vi "xboxClose.vi"() -> (0 "error out":errorcluster)   [LabVIEW 2017]
uses:
  globalDevices.vi
  <vilib>/Utility/inputDevices.llb/closeJoystick.vi
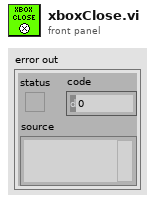
[diagram p1: front panel]
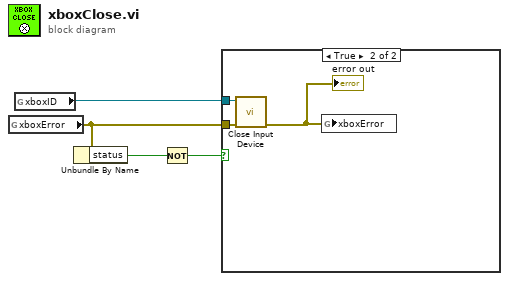
[diagram p0: block diagram]
diagram:
  n1 = global read "globalDevices.vi" "xboxError"() -> (w3:errorcluster)
  n2 = global read "globalDevices.vi" "xboxID"() -> (w4:refnum<k1>)
  n3 = Unbundle By Name(w3) -> ("status"=w2:bool)
  n4 = Not(x=w2) -> (.not. x?=w1:bool)
  n5 = case shown="True" w1 {
    tunnel: w4 -> [_ w7]
    tunnel: w3 -> [_ w5]
    frame False {
    }
    frame True {
      n6 = call-poly <vilib>:"Close Input Device.vi"("error in (no error)"=w5, "device ID"=w7) -> ("error out"=w6:errorcluster)  [unwired: 8 in]
      "error out" <- w6
      n7 = global write "globalDevices.vi" "xboxError"(w6) -> ()
    }
  }
